vi "SaveAsArrayTiff.vi"(11 "u16 array":u16[][](array[numeric])) -> ()   [LabVIEW 2018, in "RW_Protocols.lvlib"]
uses:
  RW_Protocols.lvlib
panel:
  out "error out":errorcluster
  in  "Target Folder":path
  out "selected path":path
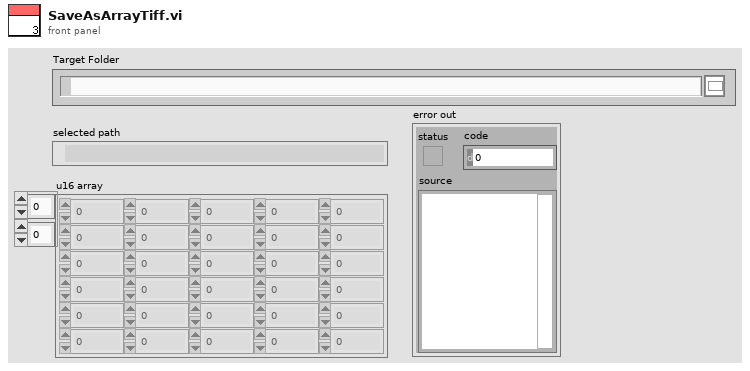
[diagram p1: front panel]
types:
  T1 = typedef "Image Type" = u32
  T2 = typedef "IMAQ Image.ctl" = refnum<image>
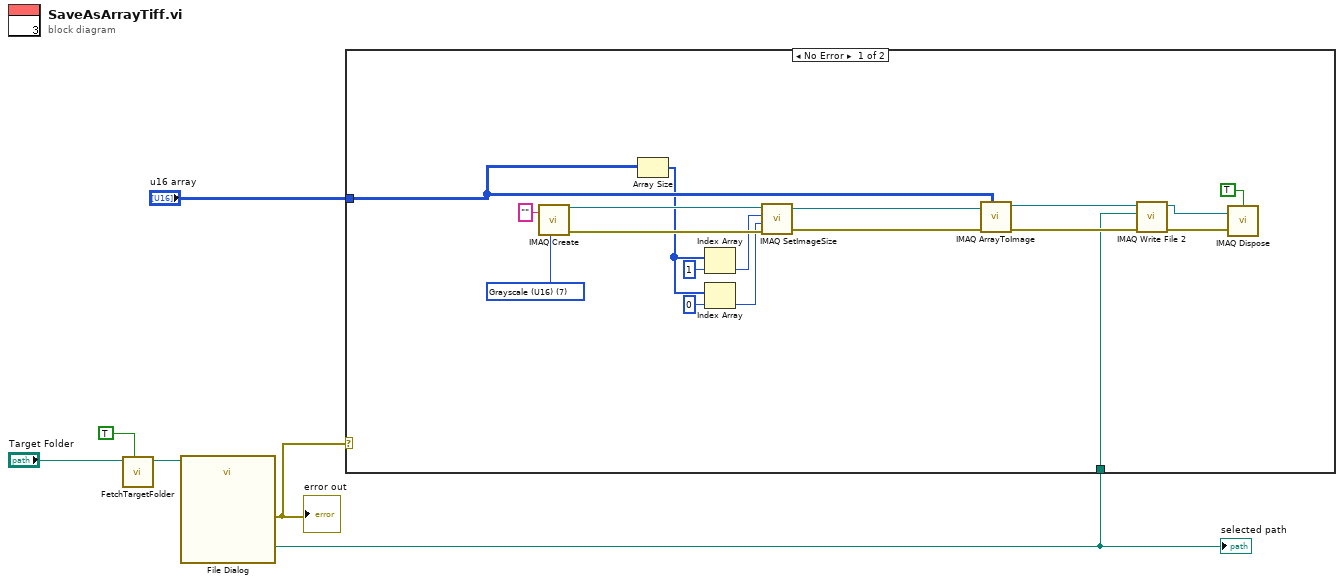
[diagram p0: block diagram]
diagram:
  n1 = call "FetchTargetFolder.vi"("Use default Folder"=TRUE, "Target Folder"="Target Folder") -> ("Full File Path"=w4:path)  [unwired: 8 in, 1 out]
  n2 = call "File Dialog"("start path"=w4) -> ("selected path"=w2:path, "error out"=w6:errorcluster)  [unwired: 11 in, 2 out]
  "selected path" <- w2
  "error out" <- w6
  n3 = case shown="No Error" w6 {
    tunnel: "u16 array" -> [w19 _]
    tunnel: w2 -> [w18 _]
    frame No Error {
      w16 = T1 7 items=["Grayscale (U8)", "Grayscale (I16)", "Grayscale (SGL)", "Complex (CSG)", "RGB (U32)", "HSL (U32)", "RGB (U64)", "Grayscale (U16)"] ("Image Type")
      n4 = call "IMAQ Create"("Image Name"="", "Image Type"=w16) -> ("New Image"=w13:T2, "error out"=w15:errorcluster)  [unwired: 3 in]
      n5 = Array Size(array=w19) -> (size(s)=w9:i32[])
      n6 = Index Array(array=w9, index=1) -> (element=w7:i32)
      n7 = Index Array(array=w9, index=0) -> (element=w10:i32)
      n8 = call "IMAQ SetImageSize"("error in (no error)"=w15, "Y Resolution"=w10, "X Resolution"=w7, "Image"=w13) -> ("error out"=w14:errorcluster, "Image Out"=w12:T2)  [unwired: 1 in]
      n9 = call "IMAQ ArrayToImage"("Image Pixels (U16)"=w19, "error in (no error)"=w14, "Image"=w12) -> ("error out"=w24:errorcluster, "Image Out"=w23:T2)  [unwired: 7 in]
      n10 = call-poly "IMAQ Write File 2"("error in (no error)"=w24, "File Path"=w18, "Image"=w23) -> ("error out"=w22:errorcluster, "Image Out (duplicate)"=w21:T2)  [unwired: 7 in]
      n11 = call "IMAQ Dispose"("All Images? (No)"=TRUE, "Image"=w21, "error in (no error)"=w22) -> ()  [unwired: 3 in, 1 out]
    }
    frame Error {
    }
  }
